vi "Disable Route.vi"(8 "error in (no error)":errorcluster, 9 "Output Index":i32, 10 "Input Index":i32, 11 "VoiceMeeterRemote in":refnum<class "VoiceMeeterRemote.lvclass">) -> (0 "error out":errorcluster, 2 "Parameter Name":string, 3 "VoiceMeeterRemote out":refnum<class "VoiceMeeterRemote.lvclass">)   [LabVIEW 2022 SP3, in "VoiceMeeterRemote.lvlib" / "VoiceMeeterRemote.lvclass"]
uses:
  VoiceMeeterRemote.lvclass
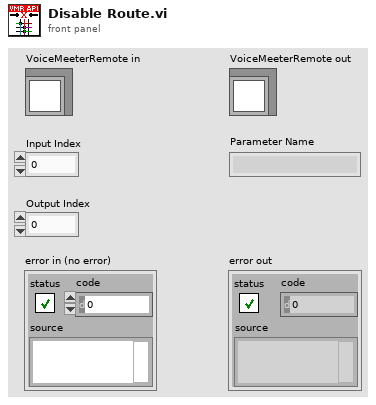
[diagram p1: front panel]
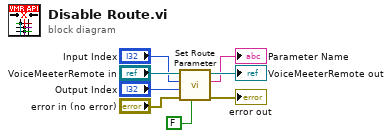
[diagram p0: block diagram]
diagram:
  n1 = call "Set Route Parameter.vi"("Connected?"=FALSE, "error in (no error)"="error in (no error)", "Output Index"="Output Index", "Input Index"="Input Index", "VoiceMeeterRemote in"="VoiceMeeterRemote in") -> ("error out"=→"error out":errorcluster, "Parameter Name"=→"Parameter Name":string, "VoiceMeeterRemote out"=→"VoiceMeeterRemote out":refnum<class "VoiceMeeterRemote.lvclass">)  [unwired: 4 in]
